vi "Property Value Updated.vi"(8 "error in":errorcluster, 10 "Property data":T1) -> (0 "error out":errorcluster)   [LabVIEW 2020, in "Plugin Template.lvlib"]
doc: "_____\nCreated using DQMH Event Scripter 6.0.0.122."
uses:
  Plugin Template.lvlib
  Property Value Updated Argument--cluster.ctl
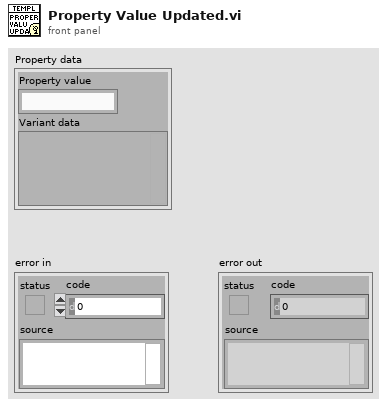
[diagram p1: front panel]
types:
  T1 = cluster{"Property value":string, "Variant data":variant}
  T2 = typedef "Plugin Template.lvlib/Property Value Updated Argument--cluster.ctl" = cluster{"Property data":cluster{"Property value":string, "Variant data":variant}}
  T3 = typedef "Plugin Template.lvlib/Broadcast Events--cluster.ctl" = cluster{"Module Did Init":refnum<user-event>, "Status Updated":refnum<user-event>, "Error Reported":refnum<user-event>, "Module Did Stop":refnum<user-event>, "Update Module Execution Status":refnum<user-event>, "Property Value Updated":refnum<user-event>}
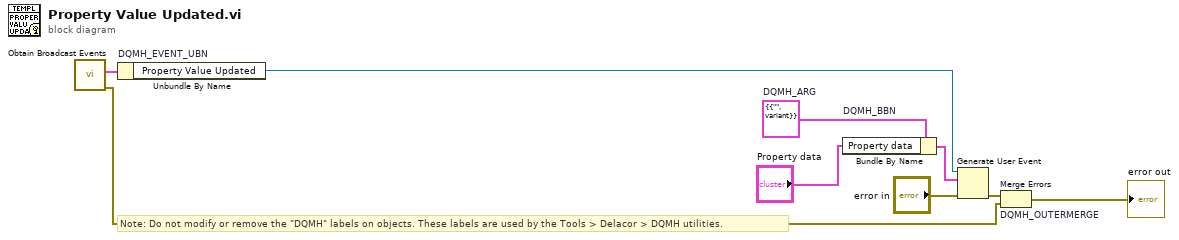
[diagram p0: block diagram]
diagram:
  w4 = T2 {"Property data"={"Property value"="", "Variant data"=variant}}  # DQMH_ARG
  # "Note: Do not modify or remove the \"DQMH\" labels on objects. These labels are used by the Tools > Delacor > DQMH utilities."
  n1 = call "Obtain Broadcast Events.vi"() -> ("error out"=w2:errorcluster, "Plugin Template Broadcast Events"=w1:T3)  [unwired: 10 in]
  n2 = Unbundle By Name "DQMH_EVENT_UBN"(w1) -> ("Property Value Updated"=w6:refnum<user-event>)
  n3 = Bundle By Name "DQMH_BBN"(cluster=w4, "Property data"="Property data") -> (w7:T2)
  n4 = Generate User Event(user event=w6, event data cluster=w7, error in="error in") -> (error out=w5:errorcluster)  [unwired: 1 in, 1 out]
  n5 = Merge Errors "DQMH_OUTERMERGE"(w5, w2) -> (→"error out":errorcluster)
